vi "LeggiDBMeta.vi"(0 "Table":refnum<vi>, 1 "raw":i32) -> ()   [LabVIEW 2018]
uses:
  D:/LIBRERIE_LV/SQLite/subvi/TypeDef/Tipo_sqlite_open.ctl
  D:/LIBRERIE_LV/SQLite/sqlite3.lvlib
panel:
  out "String":string
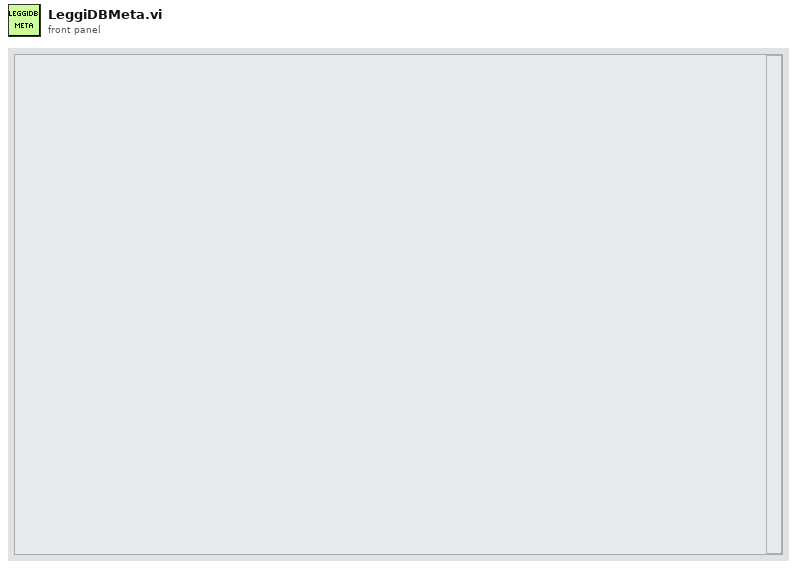
[diagram p1: front panel]
types:
  T1 = typedef "sqlite3.lvlib/Tipo_sqlite_open.ctl" = enum16{"file", "in memory"}
  T2 = cluster{"Query result[0]":string, "Query result[1]":string, "Query result[2]":string, "Query result[3]":string, "Query result[4]":string, "Query result[5]":string, "Query result[6]":string, "Query result[7]":string, "Query result[8]":string}
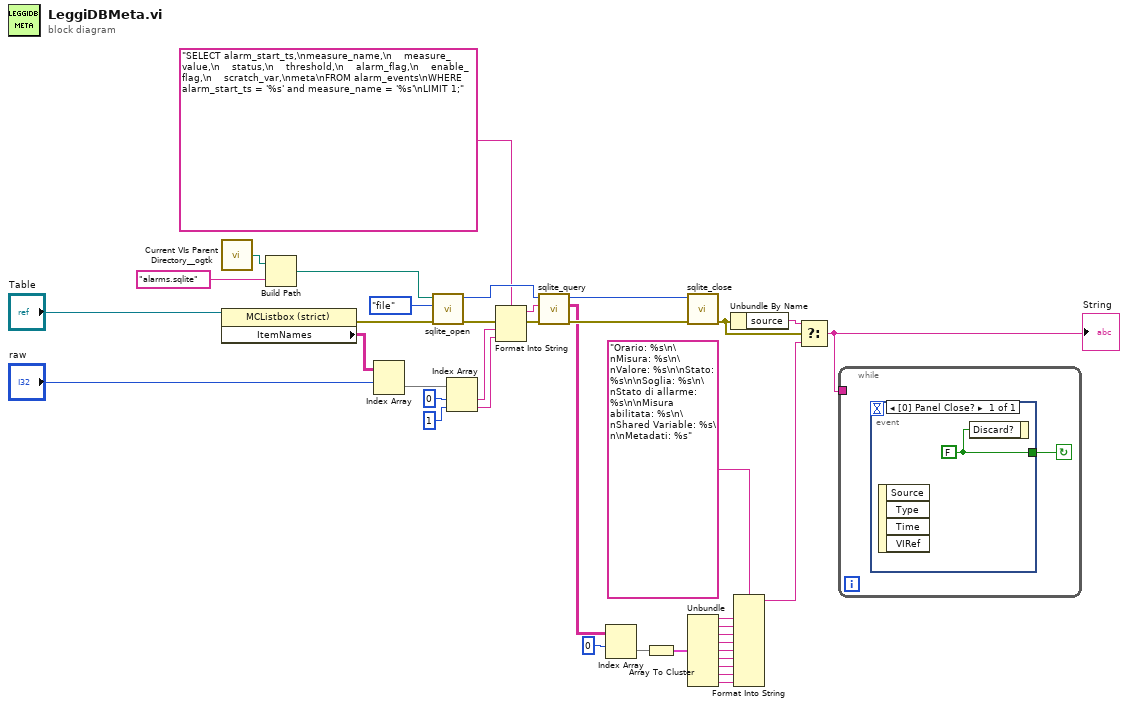
[diagram p0: block diagram]
diagram:
  n1 = call <userlib>:"Current VIs Parent Directory__ogtk.vi"() -> ("Parent Directory (+ Relative)"=w36:path)  [unwired: 5 in]
  n2 = property class="MCListbox (strict)"(reference="Table") -> (error out=w19:errorcluster, "ItemNames"=w27:string[][])  [unwired: 1 in, 1 out]
  n3 = Build Path(base path=w36, name or relative path="alarms.sqlite") -> (appended path=w35:path)
  n4 = Index Array(array=w27, index (row)="raw") -> (element=w25:string[])  [unwired: 1 in]
  n5 = call "sqlite_open.vi"("error in (no error)"=w19, "mode"=Tipo_sqlite_open."file", "Path"=w35) -> ("error out"=w30:errorcluster, "ppDb"=w38:u32)  [unwired: 7 in]
  n6 = Index Array(array=w25, index #1=0 ("index"), index #2=1 ("index")) -> (element #1=w20:string, element #2=w21:string)
  n7 = Format Into String(format string="SELECT alarm_start_ts,\nmeasure_name,\n    measure_value,\n    status,\n    threshold,\n    alarm_flag,\n    enable_flag,\n    scratch_var,\nmeta\nFROM alarm_events\nWHERE alarm_start_ts = '%s' and measure_name = '%s'\nLIMIT 1;", error in=w30, w20, w21) -> (resulting string=w31:string, error out=w29:errorcluster)  [unwired: 1 in]
  n8 = call "sqlite_query.vi"("error in (no error)"=w29, "Query"=w31, "db in"=w38) -> ("error out"=w32:errorcluster, "Query result"=w3:string[][], "db out"=w37:u32)  [unwired: 6 in]
  n9 = Index Array(array=w3, index (row)=0) -> (element=w2:string[])  [unwired: 1 in]
  n10 = Array To Cluster(array=w2) -> (cluster=w14:T2)
  n11 = call "sqlite_close.vi"("error in (no error)"=w32, "db in"=w37) -> ("error out"=w18:errorcluster)  [unwired: 9 in]
  n12 = Unbundle(w14) -> ("Query result[0]"=w13:string, "Query result[1]"=w12:string, "Query result[2]"=w11:string, "Query result[3]"=w10:string, "Query result[4]"=w9:string, "Query result[5]"=w8:string, "Query result[6]"=w7:string, "Query result[7]"=w6:string, "Query result[8]"=w5:string)
  n13 = Unbundle By Name(w18) -> ("source"=w17:string)
  n14 = Format Into String(format string="Orario: %s\n\nMisura: %s\n\nValore: %s\n\nStato: %s\n\nSoglia: %s\n\nStato di allarme: %s\n\nMisura abilitata: %s\n\nShared Variable: %s\n\nMetadati: %s", w13, w12, w11, w10, w9, w8, w7, w6, w5) -> (resulting string=w1:string)  [unwired: 2 in, 1 out]
  n15 = Select(t=w17, s=w18, f=w1) -> (s? t:f=w16:string)
  "String" <- w16
  n16 = while {
    tunnel: w16 -> [_]
    stop <- w39 continue-if-true
    n17 = event shown="[0] Panel Close?" {
      selector: _ -> [_]
      dyn-events: _ -> [_]
      timeout: _ -> [_]
      tunnel: [w40] -> w39
      event Panel Close? {
        w40 = FALSE ("Discard?")
        n18 = event-data() -> ()  [unwired: 1 in, 4 out]
        n19 = event-data("Discard?"=w40) -> ()  [unwired: 1 in, 1 out]
      }
    }
  }
